vi "rqcBob Stop.vi"(0 "rqcBob in":refnum<class "rqcBob.lvclass">, 11 "error in (no error)":errorcluster) -> (4 "rqcBob out":refnum<class "rqcBob.lvclass">, 15 "error out":errorcluster)   [LabVIEW 2018, in "rqcBob.lvclass"]
uses:
  rqcBob.lvclass
  rqcBob.lvclass/rqcBob.ctl
  Custom Controls/rqcBob State.ctl
  Custom Controls/rqcBob Main FPGA interface.ctl
  <vilib>/Utility/error.llb/Error Cluster From Error Code.vi
  <vilib>/rvi/errors/niLvFpgaAdjustHostInterfaceError.vi
  <vilib>/rvi/interface/nirviReadWriteControl/nirviReadWriteControl.xnode
  NiFpgaLv.dll
  <vilib>/rvi/interface/Simulation/niFpgaSimulationCallBeginRW.vi
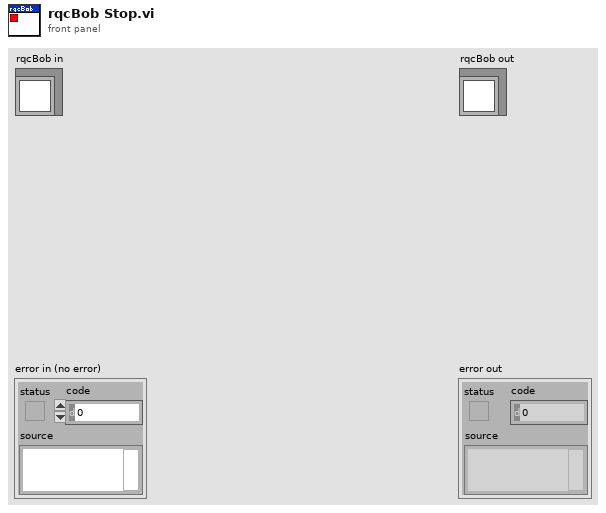
[diagram p1: front panel]
types:
  T1 = typedef "rqcBob.lvclass/rqcBob State.ctl" = enum16{"Idle", "Run"}
  T2 = typedef "rqcBob.lvclass/rqcBob Main FPGA interface.ctl" = refnum<k20>
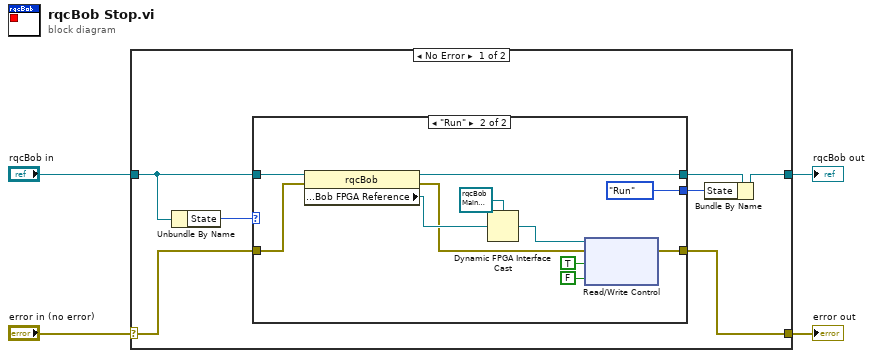
[diagram p0: block diagram]
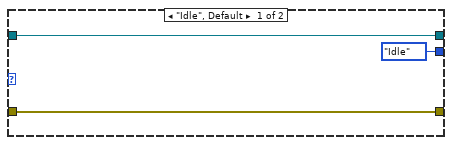
[diagram p2: hidden frame]
diagram:
  n1 = case shown="No Error" "error in (no error)" {
    selector: "error in (no error)" -> [w7 w27]
    tunnel: [w6 w27] -> w3
    tunnel: [w5 w26] -> w1
    tunnel: "rqcBob in" -> [w8 w26]
    frame No Error {
      n2 = Unbundle By Name(w8) -> ("State"=w11:T1)
      n3 = case shown="\"Run\"" w11 {
        tunnel: w8 -> [w14 w25]
        tunnel: [w14 w17] -> w10
        tunnel: w7 -> [w13 w24]
        tunnel: [w13 w16] -> w6
        tunnel: [rqcBob_State."Idle" ("State") rqcBob_State."Run" ("State")] -> w9
        frame "Idle", Default {
        }
        frame "Run" {
          n4 = property class="rqcBob"(reference=w25, error in=w24) -> (reference out=w17:refnum<class "rqcBob.lvclass">, error out=w20:errorcluster, "public:Public Properties Access:Bob FPGA Reference"=w22:refnum<k20>)
          n5 = Dynamic FPGA Interface Cast(Session In=T2 refnum ("Bob main FPGA interface"), Type=w22) -> (Session Out=w21:T2)
          n6 = xnode "Read/Write Control"("FPGA VI Reference In"=w21, "error in"=w20, "main.reset"=TRUE, "main.reset"=FALSE) -> ("error out"=w16:errorcluster)  [unwired: 1 out]
        }
      }
      n7 = Bundle By Name(cluster=w10, "State"=w9) -> (w5:refnum<class "rqcBob.lvclass">)
    }
    frame Error {
    }
  }
  "error out" <- w3
  "rqcBob out" <- w1
